vi "set output trigger period.vi"(8 "error in (no error)":errorcluster, 10 "Output trigger connector":T1=enum."3", 11 "DAQOrcaFlash in":refnum<class "DAQOrcaFlash.lvclass">) -> (0 "error out":errorcluster, 3 "DAQOrcaFlash out":refnum<class "DAQOrcaFlash.lvclass">)   [LabVIEW 2012, in "DAQOrcaFlash.lvclass"]
uses:
  DAQOrcaFlash.lvclass
  connector.ctl
  DAQOrcaFlash.lvclass/DAQOrcaFlash.ctl
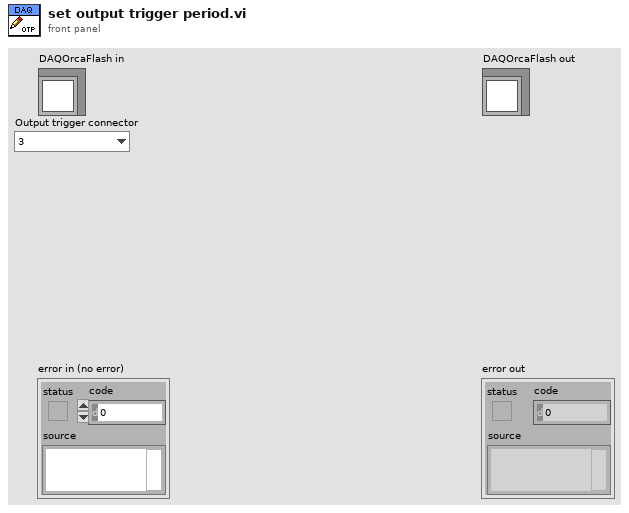
[diagram p1: front panel]
types:
  T1 = typedef "DAQOrcaFlash.lvclass/connector.ctl" = enum32{"1", "2", "3"}
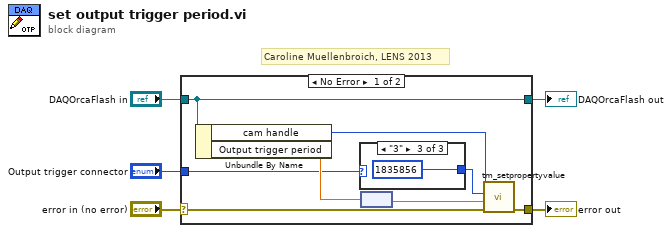
[diagram p0: block diagram]
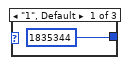
[diagram p2: hidden frame]
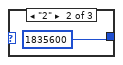
[diagram p3: hidden frame]
diagram:
  # "Caroline Muellenbroich, LENS 2013"
  n1 = case shown="No Error" "error in (no error)" {
    selector: "error in (no error)" -> [w11 w18]
    tunnel: [w10 w18] -> w4
    tunnel: [w13 w17] -> w2
    tunnel: "DAQOrcaFlash in" -> [w13 w17]
    tunnel: "Output trigger connector" -> [w6 _]
    frame No Error {
      n2 = Unbundle By Name(w13) -> ("cam handle"=w12:u32, "Output trigger period"=w9:sgl[unit])
      n3 = case shown="\"3\"" w6 {
        tunnel: [u32 1835344 ("Property ID") u32 1835600 ("Property ID") u32 1835856 ("Property ID")] -> w8
        frame "1", Default {
        }
        frame "2" {
        }
        frame "3" {
        }
      }
      n4 = node(w9) -> (w7:sgl)
      n5 = call <userlib>:"tm_setpropertyvalue.vi"("error in (no error)"=w11, "Value in"=w7, "Property ID"=w8, "Handle in"=w12) -> ("error out"=w10:errorcluster)  [unwired: 6 in, 1 out]
    }
    frame Error {
    }
  }
  "error out" <- w4
  "DAQOrcaFlash out" <- w2
